vi "Search 1D Array PtByPt.vi"(2 "initialize":bool, 3 "sample length":i32=100, 4 "element":dbl format="%0.2f", 5 "input data point":dbl format="%0.2f") -> (0 "error":i32, 1 "index":i32)   [LabVIEW 2017, in "NI_PtbyPt.lvlib"]
doc: "Searches for an element in the set of input data points specified by <B>sample length</B>."
uses:
  <vilib>/ptbypt/NI_PtbyPt.lvlib
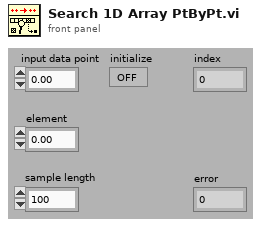
[diagram p1: front panel]
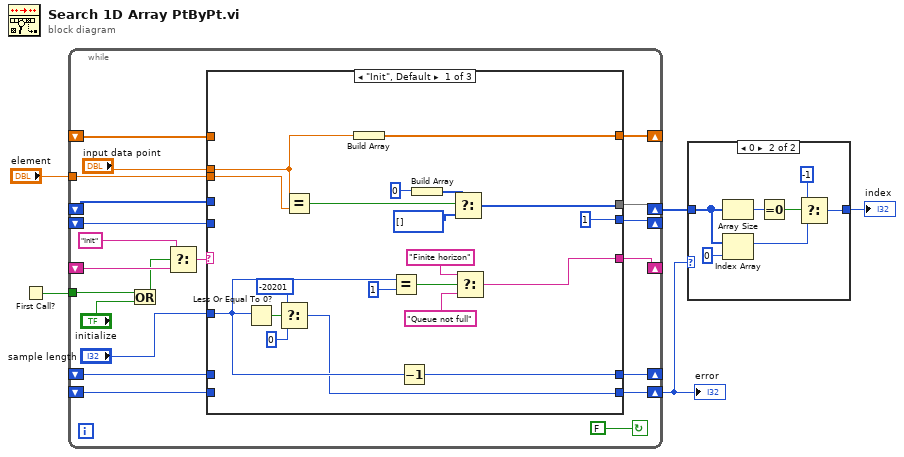
[diagram p0: block diagram]
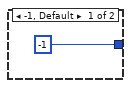
[diagram p2: hidden frame]
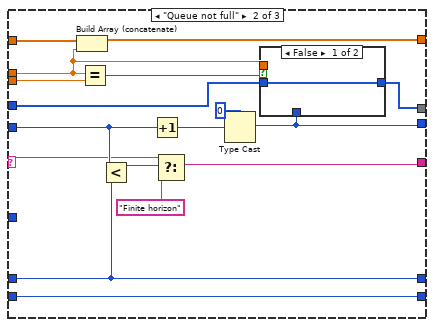
[diagram p3: hidden frame]
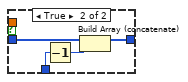
[diagram p4: hidden frame]
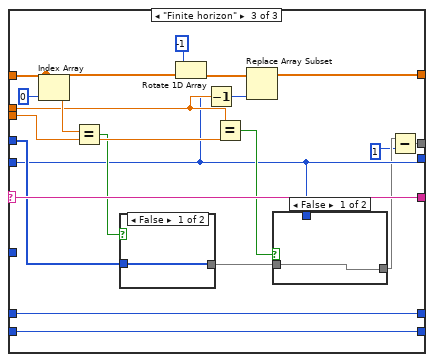
[diagram p5: hidden frame]
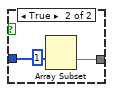
[diagram p6: hidden frame]
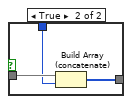
[diagram p7: hidden frame]
diagram:
  n1 = First Call?() -> (First Call?: T/F=w2:bool)
  n2 = while {
    shift-left: _ -> [w8]
    shift-right: [w9] -> _
    tunnel: w2 -> [w12]
    shift-left: _ -> [w16]
    shift-right: [w17] -> w4
    tunnel: "element" -> [w18]
    shift-left: _ -> [w20]
    shift-right: [w19] -> _
    shift-left: _ -> [w22]
    shift-right: [w23] -> _
    shift-left: _ -> [w26]
    shift-right: [w21] -> _
    shift-right: [w7] -> w1
    shift-left: _ -> [w6]
    stop <- FALSE continue-if-true
    n3 = Or(x=w12, y="initialize") -> (x .or. y?=w10:bool)
    n4 = Select(t="Init", s=w10, f=w26) -> (s? t:f=w24:string)
    n5 = case shown="\"Init\", Default" w24 {
      selector: w24 -> [_ w57 w82]
      tunnel: "input data point" -> [w36 w52 w75]
      tunnel: [1 w50 w74] -> w23
      tunnel: w22 -> [_ w59 w74]
      tunnel: [w38 w55 w82] -> w21
      tunnel: w20 -> [_ w63 w83]
      tunnel: [w33 w62 w84] -> w19
      tunnel: "sample length" -> [w29 _ _]
      tunnel: w18 -> [w37 w54 w79]
      tunnel: [w34 w49 w73] -> w17
      tunnel: w16 -> [_ w51 w77]
      tunnel: [w28 w48 w70] -> w9
      tunnel: w8 -> [_ w48 w70]
      tunnel: [w27 w47 w69] -> w7
      tunnel: w6 -> [_ w47 w69]
      frame "Init", Default {
        n6 = Less Or Equal To 0?(x=w29) -> (x <= 0?=w39:bool)
        n7 = Select(t=-20201, s=w39, f=0) -> (s? t:f=w27:i32)
        n8 = Equal?(x=w36, y=w37) -> (x = y?=w35:bool)
        n9 = Build Array(w36) -> (w33:dbl[])
        n10 = Equal?(x=w29, y=1) -> (x = y?=w44:bool)
        n11 = Decrement(x=w29) -> (x-1=w28:i32)
        n12 = Build Array(0) -> (w32:i32[])
        n13 = Select(t=w32, s=w35, f=i32[] []) -> (s? t:f=w34:i32[])
        n14 = Select(t="Finite horizon", s=w44, f="Queue not full") -> (s? t:f=w38:string)
      }
      frame "Queue not full" {
        n15 = Build Array (concatenate)(w63, w52) -> (w62:dbl[])
        n16 = Equal?(x=w52, y=w54) -> (x = y?=w53:bool)
        n17 = Less?(x=w59, y=w48) -> (x < y?=w58:bool)
        n18 = Increment(x=w59) -> (x+1=w61:i32)
        n19 = Select(t=w57, s=w58, f="Finite horizon") -> (s? t:f=w55:string)
        n20 = Type Cast(type=0, x=w61) -> (*(type *) &x=w50:i32)
        n21 = case shown="False" w53 {
          tunnel: w51 -> [w64 w68]
          tunnel: w52 -> [_ _]
          tunnel: w50 -> [_ w67]
          tunnel: [w64 w66] -> w49
          frame False {
          }
          frame True {
            n22 = Decrement(x=w67) -> (x-1=w65:i32)
            n23 = Build Array (concatenate)(w68, w65) -> (w66:i32[])
          }
        }
      }
      frame "Finite horizon" {
        n24 = Index Array(array=w83, index=0 ("Index")) -> (element=w80:dbl)
        n25 = Equal?(x=w80, y=w79) -> (x = y?=w78:bool)
        n26 = case shown="False" w78 {
          tunnel: w77 -> [w89 w92]
          tunnel: [w89 w90] -> w76
          frame False {
          }
          frame True {
            n27 = Array Subset(array=w92, index=1 ("Array Index")) -> (w90:i32[])  [unwired: 1 in]
          }
        }
        n28 = Rotate 1D Array(1:w83, 2:i16 -1 ("n")) -> (0:w86:dbl[])
        n29 = Decrement(x=w74) -> (x-1=w85:i32)
        n30 = Equal?(x=w75, y=w79) -> (x = y?=w81:bool)
        n31 = Replace Array Subset(array=w86, new element=w75, index=w85) -> (w84:dbl[])
        n32 = case shown="False" w81 {
          tunnel: w76 -> [w93 w96]
          tunnel: [w93 w95] -> w72
          tunnel: w74 -> [_ w94]
          frame False {
          }
          frame True {
            n33 = Build Array (concatenate)(w96, w94) -> (w95:i32[])
          }
        }
        n34 = Subtract(x=w72, y=1) -> (x-y=w73:i32[])
      }
    }
  }
  "error" <- w1
  n35 = case shown="0" w1 {
    tunnel: w4 -> [_ w101]
    tunnel: [-1 w98] -> w3
    frame -1, Default {
    }
    frame 0 {
      n36 = Array Size(array=w101) -> (size(s)=w104:i32)
      n37 = Index Array(array=w101, index=0 ("Index")) -> (element=w100:i32)
      n38 = Equal To 0?(x=w104) -> (x = 0?=w103:bool)
      n39 = Select(t=-1, s=w103, f=w100) -> (s? t:f=w98:i32)
    }
  }
  "index" <- w3
